vi "Load Control (Path).vi"(8 "error in (no error)":errorcluster, 10 "Path":path, 11 "Control List in":refnum<class "Control List.lvclass">) -> (0 "error out":errorcluster, 3 "Control List out":refnum<class "Control List.lvclass">)   [LabVIEW 2020, in "VolatusGUIEditor.lvlib" / "Control List.lvclass"]
uses:
  Control List.lvclass
  Control List.lvclass/Control List.ctl
  VolatusGUIEditor.lvlib
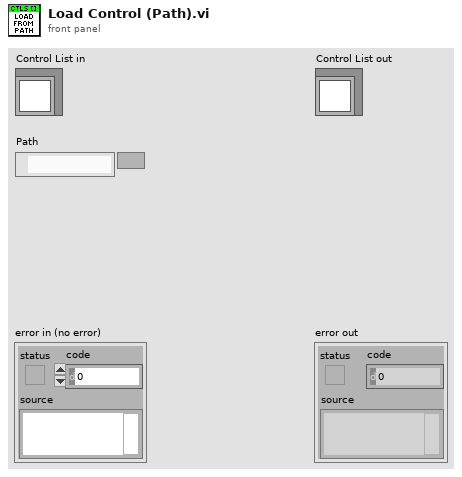
[diagram p1: front panel]
types:
  T1 = typedef "VolatusGUIEditor.lvlib/Control Info.ctl" = cluster{"Description":string, "Hierarchy":string[], "Image":T2, "Element Type":string}
  T2 = typedef "imagedata.ctl" = cluster{"image type":i32, "image depth":i32, "image":u8[], "mask":u8[], "colors":u32[], "Rectangle":cluster{"left":i16, "top":i16, "right":i16, "bottom":i16}}
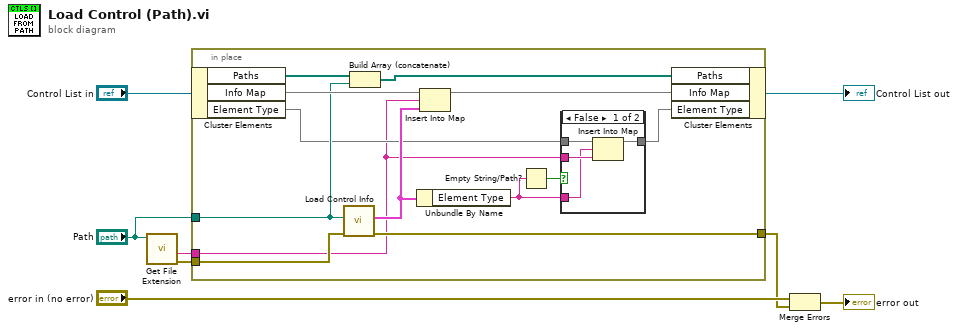
[diagram p0: block diagram]
diagram:
  n1 = call <vilib>:"Get File Extension.vi"("file"="Path") -> ("error out"=w3:errorcluster, "filename without extension"=w5:string)  [unwired: 6 in, 3 out]
  n2 = in-place {
    in-place-border: w5 -> [w10]
    in-place-border: "Path" -> [w18]
    in-place-border: w3 -> [w20]
    in-place-border: [w15] -> w1
    n3 = in-place-cluster #1("Control List in") -> ("Paths"=w21:path[], "Info Map"=w19:map{string, T1}, "Element Type"=w11:map{string, string})
    n4 = call "Load Control Info.vi"("error in (no error)"=w20, "Control Path"=w18) -> ("error out"=w15:errorcluster, "Info"=w14:T1)  [unwired: 8 in]
    n5 = Build Array (concatenate)(w21, w18) -> (w17:path[])
    n6 = Unbundle By Name(w14) -> ("Element Type"=w12:string)
    n7 = Insert Into Map(map in=w19, key=w10, value=w14) -> (map out=w16:map{string, T1})  [unwired: 2 out]
    n8 = Empty String/Path?(string/path=w12) -> (empty?=w13:bool)
    n9 = case shown="False" w13 {
      tunnel: w12 -> [w23 _]
      tunnel: w11 -> [w25 w26]
      tunnel: w10 -> [w24 _]
      tunnel: [w22 w26] -> w9
      frame False {
        n10 = Insert Into Map(map in=w25, key=w23, value=w24) -> (map out=w22:map{string, string})  [unwired: 2 out]
      }
      frame True {
      }
    }
    n11 = in-place-cluster #1("Paths"=w17, "Info Map"=w16, "Element Type"=w9) -> (→"Control List out":refnum<class "Control List.lvclass">)
  }
  n12 = Merge Errors("error in (no error)", w1) -> (→"error out":errorcluster)
